vi "StudyAOSettling.vi"() -> ()   [LabVIEW 2014]
doc: "Use this template to build a user interface event handler design pattern. Use this pattern for dialog boxes and other user interfaces. You also can create and execute user-defined events that the VI can handle the same way as user interface events."
panel:
  out "Approx. Slew Rate":dbl format="%#_3p"
  out "Settling Time":dbl format="%#_3p"
  in  "Signal Generation":T1={"Signal Type"=enum."Sine Wave", "Amplitude"=5.0, "Frequency"=1000.0} {"Frequency" format="%.2p"; "Amplitude" format="%0.2p"}
  in  "Timing":cluster{"Sample Rate":dbl, "Duration":dbl}={"Sample Rate"=200000.0, "Duration"=1.0} {"Duration" format="%#_3p"; "Sample Rate" format="%#_3p"}
  in  "Output":T2={"Channel"="myDAQ1/ao0", "Minimum Value"=-10.0, "Maximum Value"=10.0}
  in  "Input":T2={"Channel"="myDAQ1/ai0", "Minimum Value"=-2.0, "Maximum Value"=2.0}
  out "Waveform Graph":waveform(dbl)(graph)
  in  "Go":bool
  in  "stop":bool
  # "s"
  # "V/s"
  # "Hz"
  # "V"
  # "Hz"
  # "s"
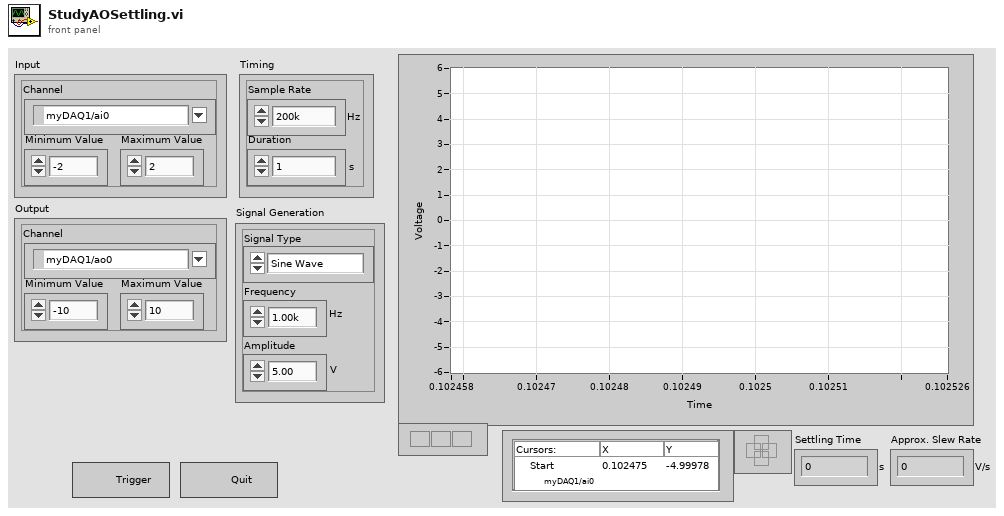
[diagram p1: front panel]
types:
  T1 = cluster{"Signal Type":enum16{"Sine Wave", "Triangle Wave", "Square Wave", "Sawtooth Wave"}, "Amplitude":dbl, "Frequency":dbl}
  T2 = cluster{"Channel":tag, "Minimum Value":dbl, "Maximum Value":dbl}
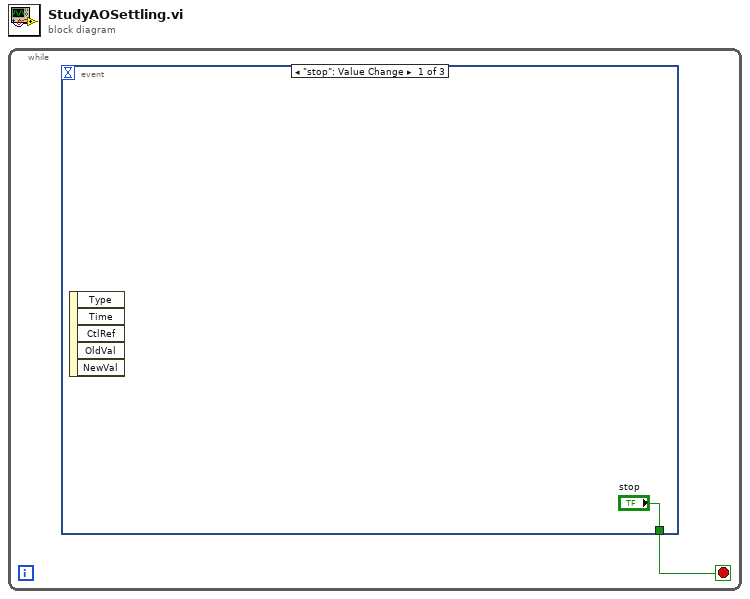
[diagram p0: block diagram]
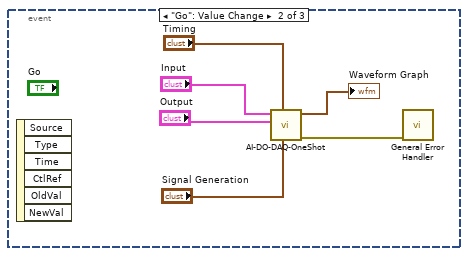
[diagram p2: hidden frame]
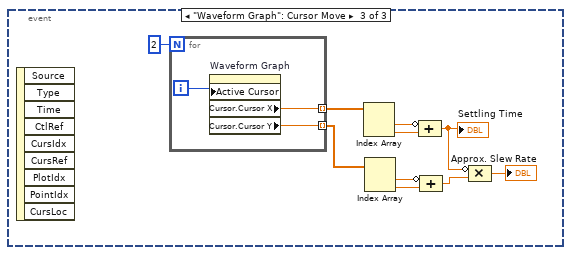
[diagram p3: hidden frame]
diagram:
  n1 = while {
    stop <- w1 stop-if-true
    n2 = event shown="[0] \"stop\": Value Change" {
      selector: _ -> [_ _ _]
      dyn-events: _ -> [_ _ _]
      timeout: _ -> [_ _ _]
      tunnel: ["stop" _ _] -> w1
      event "stop": Value Change {
        n3 = event-data() -> ()  [unwired: 1 in, 5 out]
      }
      event "Go": Value Change {
        n4 = event-data() -> ()  [unwired: 1 in, 6 out]
        n5 = call "AI-DO-DAQ-OneShot.vi"("Signal Generation"="Signal Generation", "Timing Parameters"="Timing", "Output"="Output", "Input"="Input") -> ("error out"=w3:errorcluster, "Measurement"=→"Waveform Graph":waveform(dbl))  [unwired: 5 in, 1 out]
        n6 = call <vilib>:"General Error Handler.vi"("error in (no error)"=w3) -> ()  [unwired: 10 in, 5 out]
      }
      event "Waveform Graph": Cursor Move {
        n7 = event-data() -> ()  [unwired: 1 in, 9 out]
        n8 = for {
          N: 2 -> [_]
          tunnel: [w20] -> w17 mode=indexing
          tunnel: [w19] -> w12 mode=indexing
          i -> [w21]
          n9 = property on="Waveform Graph" class="WFGraph (strict)"("Active Cursor"=w21) -> ("Cursor.Cursor X"=w20:dbl, "Cursor.Cursor Y"=w19:dbl)  [unwired: 2 in, 2 out]
        }
        n10 = Index Array(array=w17) -> (element #1=w15:dbl, element #2=w16:dbl)  [unwired: 2 in]
        n11 = Index Array(array=w12) -> (element #1=w14:dbl, element #2=w13:dbl)  [unwired: 2 in]
        n12 = Compound Arithmetic op=ADD(invert w15, w16) -> (w11:dbl)
        "Settling Time" <- w11
        n13 = Compound Arithmetic op=ADD(invert w14, w13) -> (w10:dbl)
        n14 = Compound Arithmetic op=MULTIPLY(invert w11, w10) -> (→"Approx. Slew Rate":dbl)
      }
    }
  }
